vi "Build Picture JSON.vi"(8 "error in (no error)":errorcluster, 11 "<JSON> in":string) -> (0 "error out":errorcluster, 3 "<JSON> out":string)   [LabVIEW 2025, in "MCP Server.lvlib"]
uses:
  MCP Server.lvlib
  a662b823-3d79-4c18-8875-22636ac4371e.vi
  <vilib>/JDP Science/JSONtext/Variant to JSON Text.vi
  <vilib>/JDP Science/JSONtext/LVClass Serializer/JSONtext LVClass Serializer.lvclass
  <vilib>/JDP Science/JSONtext/JSONtext.lvlib
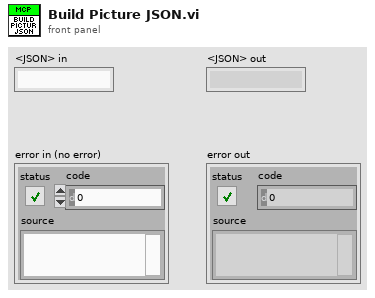
[diagram p1: front panel]
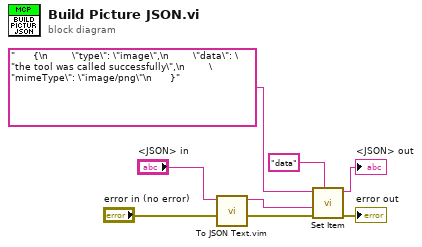
[diagram p0: block diagram]
diagram:
  n1 = call "To JSON Text.vim"("error in (no error)"="error in (no error)", "Anything"="<JSON> in") -> ("error out"=w7:errorcluster, "<JSON>"=w5:string)  [unwired: 8 in]
  n2 = call <vilib>:"Set Item.vi"("$Path or Item Name"="data", "error in (no error)"=w7, "JSON to Insert"=w5, "JSON"="      {\n        \"type\": \"image\",\n        \"data\": \"the tool was called successfully\",\n        \"mimeType\": \"image/png\"\n      }" ("element")) -> ("error out"=→"error out":errorcluster, "<JSON>"=→"<JSON> out":string)  [unwired: 4 in, 1 out]
